vi "send&receive_multy_arrs.vi"() -> ()   [LabVIEW 2018, in "LV-Julia_ZMQ-Roundtrip_lib.lvlib"]
uses:
  LV-Julia_ZMQ-Roundtrip_lib.lvlib
  Server or client state.ctl
  detailed error info.ctl
  StackFrame.ctl
  Commands v2.ctl
  commands LV2Jl.ctl
  Julia functions enum.ctl
  0f3c6ff9-6efb-4048-9743-f0faf74ba571.vi
  1180a24e-9cfc-4814-956e-56f85e4fc15d.vi
  d2cb43a9-9305-42fb-ad58-bce983510195.vi
  4837e4b1-53a7-49b6-9aef-263877b89a45.vi
  5398bb44-7854-4704-a5a4-70900ab1788b.vi
  0f3c6ff9-6efb-4048-9743-f0faf74ba571.vi/a8133a9d-5cb4-4f45-826d-93f84bf6eb0d.vi
  0f3c6ff9-6efb-4048-9743-f0faf74ba571.vi/13f44d60-32a4-4ee7-b81c-21f7a391c3aa.vi
  0f3c6ff9-6efb-4048-9743-f0faf74ba571.vi/9f4fcee5-9fb3-4ec4-aeb1-d194e55cfefe.vi
  0f3c6ff9-6efb-4048-9743-f0faf74ba571.vi/1d479851-527b-4588-bf0b-60628e8bf317.vi
  0f3c6ff9-6efb-4048-9743-f0faf74ba571.vi/26ca6034-af2a-482b-8391-d55ce4957874.vi
  1180a24e-9cfc-4814-956e-56f85e4fc15d.vi/745acb1a-d655-4255-af81-9cf684133840.vi
  1180a24e-9cfc-4814-956e-56f85e4fc15d.vi/00973f5a-5f23-4306-b9aa-355ac52cfc45.vi
  1180a24e-9cfc-4814-956e-56f85e4fc15d.vi/c6eed95d-99c6-43df-958f-043b05f188e9.vi
  1180a24e-9cfc-4814-956e-56f85e4fc15d.vi/2e50c6a9-e645-434a-9e40-f73025a6ffce.vi
  1180a24e-9cfc-4814-956e-56f85e4fc15d.vi/339e4087-309e-456a-ab9d-330082cc7581.vi
  d2cb43a9-9305-42fb-ad58-bce983510195.vi/19be6d5a-1807-40f3-bdbe-1f3f52c696f0.vi
  d2cb43a9-9305-42fb-ad58-bce983510195.vi/aa24d0ac-04a8-4d7b-8f99-439a812d7bff.vi
  d2cb43a9-9305-42fb-ad58-bce983510195.vi/183daee5-84c7-4d39-a056-e1aa05b2b19e.vi
  4837e4b1-53a7-49b6-9aef-263877b89a45.vi/b7e14757-1b30-45b6-9c9e-f3055ae305b8.vi
  4837e4b1-53a7-49b6-9aef-263877b89a45.vi/187a7c1e-07ba-4c8d-9bdb-654d6cd0a580.vi
  5398bb44-7854-4704-a5a4-70900ab1788b.vi/24b2726a-72e9-4d38-b333-142c4ad70cae.vi
  5398bb44-7854-4704-a5a4-70900ab1788b.vi/ae670f7e-6490-4d67-937f-e0119a307e5a.vi
  0f3c6ff9-6efb-4048-9743-f0faf74ba571.vi/13f44d60-32a4-4ee7-b81c-21f7a391c3aa.vi/4fd0da60-a885-4f86-950c-51bd87ce8b7e.vi
  0f3c6ff9-6efb-4048-9743-f0faf74ba571.vi/9f4fcee5-9fb3-4ec4-aeb1-d194e55cfefe.vi/0c7f0749-4fca-4eec-9bb8-54480ed85867.vi
  0f3c6ff9-6efb-4048-9743-f0faf74ba571.vi/1d479851-527b-4588-bf0b-60628e8bf317.vi/c34eabd0-0321-4a17-ad95-65fcb7b0333a.vi
  1180a24e-9cfc-4814-956e-56f85e4fc15d.vi/00973f5a-5f23-4306-b9aa-355ac52cfc45.vi/cb92420a-3b20-40fb-957b-d1dd647802a0.vi
  1180a24e-9cfc-4814-956e-56f85e4fc15d.vi/c6eed95d-99c6-43df-958f-043b05f188e9.vi/f2a235e6-0b9e-43b4-b57c-a299a1c981e2.vi
  1180a24e-9cfc-4814-956e-56f85e4fc15d.vi/2e50c6a9-e645-434a-9e40-f73025a6ffce.vi/335e82b0-2764-49f6-958b-454fe2620a9a.vi
  4837e4b1-53a7-49b6-9aef-263877b89a45.vi/b7e14757-1b30-45b6-9c9e-f3055ae305b8.vi/13c95251-aaf3-4968-a2b1-71e97477a335.vi
  4837e4b1-53a7-49b6-9aef-263877b89a45.vi/b7e14757-1b30-45b6-9c9e-f3055ae305b8.vi/ab4a86bb-797d-4947-b82b-ab2adb434181.vi
  5398bb44-7854-4704-a5a4-70900ab1788b.vi/24b2726a-72e9-4d38-b333-142c4ad70cae.vi/167f8237-5b23-4042-87d7-597a2036b2c1.vi
  5398bb44-7854-4704-a5a4-70900ab1788b.vi/24b2726a-72e9-4d38-b333-142c4ad70cae.vi/addd60ed-eb33-4fa9-8646-f27a66fb9797.vi
  0f3c6ff9-6efb-4048-9743-f0faf74ba571.vi/13f44d60-32a4-4ee7-b81c-21f7a391c3aa.vi/4fd0da60-a885-4f86-950c-51bd87ce8b7e.vi/d91722bc-760f-488b-93ae-5bc6f1881f78.vi
  0f3c6ff9-6efb-4048-9743-f0faf74ba571.vi/9f4fcee5-9fb3-4ec4-aeb1-d194e55cfefe.vi/0c7f0749-4fca-4eec-9bb8-54480ed85867.vi/2bfc81f1-cfb7-4819-b1bc-540959743fb2.vi
  0f3c6ff9-6efb-4048-9743-f0faf74ba571.vi/1d479851-527b-4588-bf0b-60628e8bf317.vi/c34eabd0-0321-4a17-ad95-65fcb7b0333a.vi/b4dec757-f14e-4c32-8f18-a6a53eb12cfa.vi
  1180a24e-9cfc-4814-956e-56f85e4fc15d.vi/00973f5a-5f23-4306-b9aa-355ac52cfc45.vi/cb92420a-3b20-40fb-957b-d1dd647802a0.vi/e8ebe7f7-f03d-49ec-9fb8-d4a1a45a4ade.vi
  1180a24e-9cfc-4814-956e-56f85e4fc15d.vi/c6eed95d-99c6-43df-958f-043b05f188e9.vi/f2a235e6-0b9e-43b4-b57c-a299a1c981e2.vi/36ca0de6-0589-4a03-972d-fca6fdad2387.vi
  1180a24e-9cfc-4814-956e-56f85e4fc15d.vi/2e50c6a9-e645-434a-9e40-f73025a6ffce.vi/335e82b0-2764-49f6-958b-454fe2620a9a.vi/0d9d3acc-8ad3-4eff-83fb-bef53c6a881b.vi
  4837e4b1-53a7-49b6-9aef-263877b89a45.vi/b7e14757-1b30-45b6-9c9e-f3055ae305b8.vi/13c95251-aaf3-4968-a2b1-71e97477a335.vi/50b08b95-f687-4883-9b5c-2995c4691fc2.vi
  5398bb44-7854-4704-a5a4-70900ab1788b.vi/24b2726a-72e9-4d38-b333-142c4ad70cae.vi/167f8237-5b23-4042-87d7-597a2036b2c1.vi/0c43e3ab-dc7e-44be-9e5a-46602dd1e47d.vi
  0f3c6ff9-6efb-4048-9743-f0faf74ba571.vi/13f44d60-32a4-4ee7-b81c-21f7a391c3aa.vi/4fd0da60-a885-4f86-950c-51bd87ce8b7e.vi/d91722bc-760f-488b-93ae-5bc6f1881f78.vi/81bb06db-bbc8-4c4f-bf8c-0a9139f35f47.vi
  0f3c6ff9-6efb-4048-9743-f0faf74ba571.vi/9f4fcee5-9fb3-4ec4-aeb1-d194e55cfefe.vi/0c7f0749-4fca-4eec-9bb8-54480ed85867.vi/2bfc81f1-cfb7-4819-b1bc-540959743fb2.vi/ceb014c5-17c5-4aee-87b4-bdb5202f11bf.vi
  0f3c6ff9-6efb-4048-9743-f0faf74ba571.vi/1d479851-527b-4588-bf0b-60628e8bf317.vi/c34eabd0-0321-4a17-ad95-65fcb7b0333a.vi/b4dec757-f14e-4c32-8f18-a6a53eb12cfa.vi/3b214c27-556c-42a7-8fef-6ab7ffc3abfe.vi
  1180a24e-9cfc-4814-956e-56f85e4fc15d.vi/00973f5a-5f23-4306-b9aa-355ac52cfc45.vi/cb92420a-3b20-40fb-957b-d1dd647802a0.vi/e8ebe7f7-f03d-49ec-9fb8-d4a1a45a4ade.vi/a50604c4-b02c-41aa-8651-ec1557e36820.vi
  1180a24e-9cfc-4814-956e-56f85e4fc15d.vi/c6eed95d-99c6-43df-958f-043b05f188e9.vi/f2a235e6-0b9e-43b4-b57c-a299a1c981e2.vi/36ca0de6-0589-4a03-972d-fca6fdad2387.vi/17266f24-6c92-4fe0-b395-2dcbb4c32836.vi
  1180a24e-9cfc-4814-956e-56f85e4fc15d.vi/2e50c6a9-e645-434a-9e40-f73025a6ffce.vi/335e82b0-2764-49f6-958b-454fe2620a9a.vi/0d9d3acc-8ad3-4eff-83fb-bef53c6a881b.vi/8f1dd33f-3a61-4420-ad07-afe7428103ca.vi
  check ID validity.vi
  bindata_descr to JSON.vi
  convert Jl functions enum to string.vi
  check cluster field names.vi
  concat JSON.vi
  <vilib>/Utility/error.llb/Error Cluster From Error Code.vi
panel:
  out "U64arr":u64[](array[numeric])
  out "arrays equal":bool
  out "elems equal":bool
  in  "next":bool
  in  "stop LV only":bool
  in  "stop":bool
  out "detailed error info":T1
  out "elem sent":sgl
  out "elem received":dbl
  out "testarr":sgl[][](array[numeric])
  in  "index to return":cluster{"idx":u16[]}={"idx"=[3, 4, 1]} {"idx" min=1}
  out "Jl Server state out":T3
  out "short err code":u8
  out "final error":errorcluster
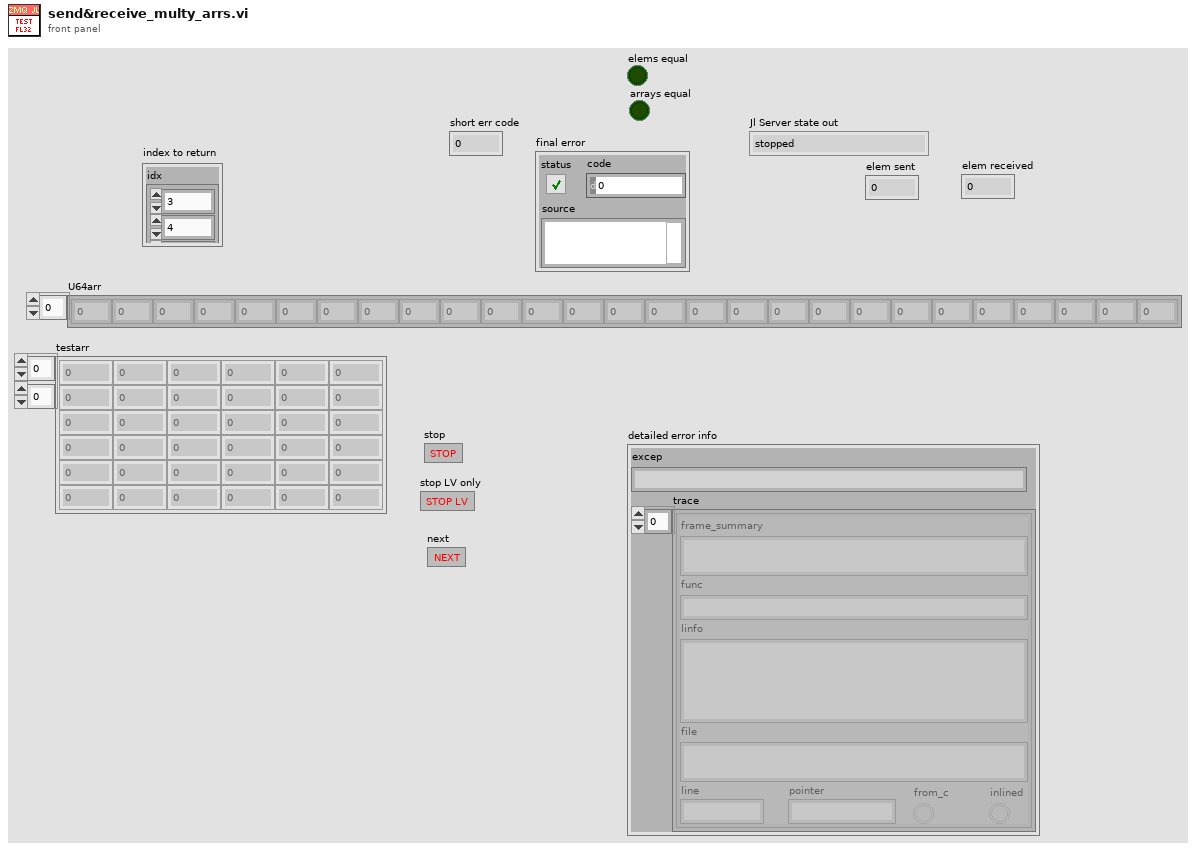
[diagram p1: front panel]
types:
  T1 = typedef "LV-Julia_ZMQ-Roundtrip_lib.lvlib/detailed error info.ctl" = cluster{"excep":string, "trace":T2[]}
  T2 = typedef "LV-Julia_ZMQ-Roundtrip_lib.lvlib/StackFrame.ctl" = cluster{"frame_summary":string, "func":string, "linfo":string, "file":string, "line":i32, "pointer":u64, "from_c":bool, "inlined":bool}
  T3 = typedef "LV-Julia_ZMQ-Roundtrip_lib.lvlib/Server or client state.ctl" = enum16{"stopped", "running", "unknown"}
  T4 = typedef "LV-Julia_ZMQ-Roundtrip_lib.lvlib/Commands v2.ctl" = enum16{"Start Jl-server & Init LV-client", "Send request & Get response ", "Stop Jl-server & Cleanup LV-client", "Cleanup LV-client", "Start Jl-server", "Stop Jl-server", "Init LV-Client", "Cleanup LV-Client", "(not allowed)", "Set LV Client state", "Set Jl Server state"}
  T5 = typedef "LV-Julia_ZMQ-Roundtrip_lib.lvlib/Julia functions enum.ctl" = enum16{"myf1", "myf2", "myf3", "test_bin2nums", "test_rgbimg", "numarr_loopback", "numarrs_lpbk", "Not_a_Fun"}
  T6 = typedef "commands LV2Jl.ctl" = u8
  T7 = typedef "Bindata&description.ctl" = cluster{"bindata_descr":T8[], "bindata":u8[]}
  T8 = typedef "LV-Julia_ZMQ-Roundtrip_lib.lvlib/Bindata description.ctl" = cluster{"nofbytes":i32, "numtype":string, "start":i32, "arrdims":i32[], "kwarg_name":string, "category":string}
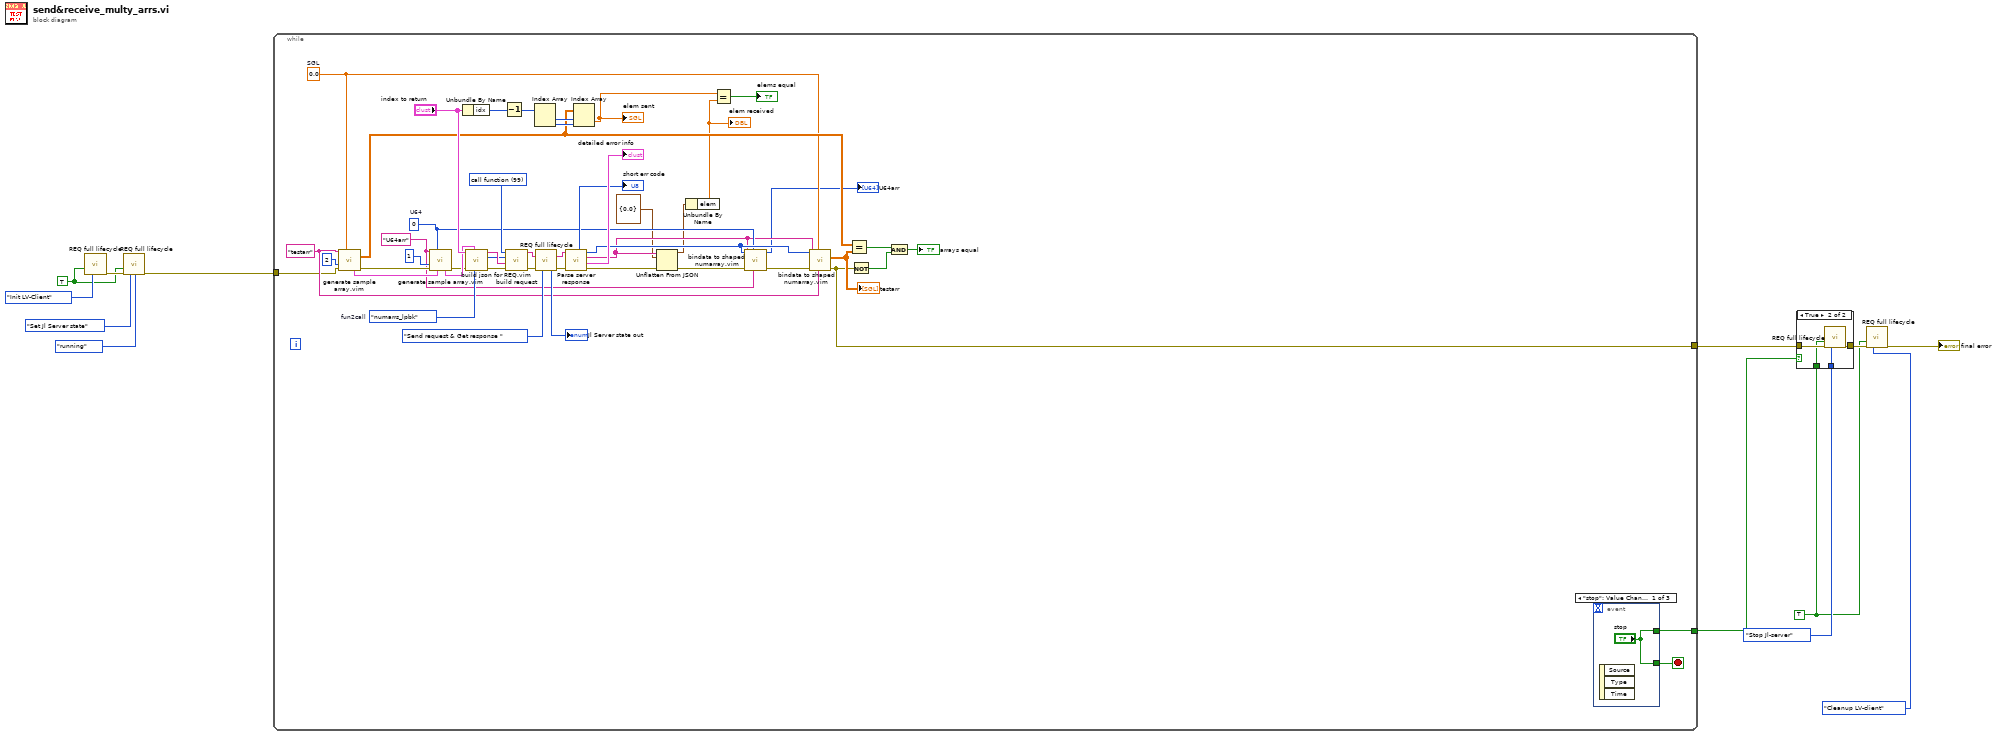
[diagram p0: block diagram]
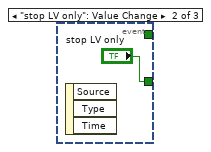
[diagram p2: hidden frame]
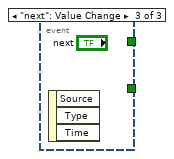
[diagram p3: hidden frame]
diagram:
  w4 = TRUE ("Force command")
  w8 = TRUE ("Force command")
  n1 = call "REQ full lifecycle.vi"("Force command"=w4, "command"=Commands_v2."Init LV-Client") -> ("error out"=w6:errorcluster)  [unwired: 10 in, 3 out]
  n2 = call "REQ full lifecycle.vi"("Force command"=w4, "error in"=w6, "command"=Commands_v2."Set Jl Server state", "Jl Server state in"=Server_or_client_state."running") -> ("error out"=w2:errorcluster)  [unwired: 8 in, 3 out]
  n3 = while {
    tunnel: w2 -> [w40]
    tunnel: [w32] -> w13
    tunnel: [w35] -> w1
    stop <- w36 stop-if-true
    w19 = "U64arr" ("kwarg_name")
    w21 = u64 0  # U64
    w29 = sgl 0.0  # SGL
    w54 = Julia_functions_enum."numarrs_lpbk"  # fun2call
    w47 = "testarr" ("Tag")
    w55 = T6 99 items=["call function"=99, "ping"=112, "stop"=115] ("Command")
    n4 = call "generate sample array.vim"("kwarg_name"=w47, "type"=w29, "dims"=2 ("arr1 dimension"), "error in (no error)"=w40) -> ("Array 2D"=w31:sgl[][], "Bindata & descr out"=w28:T7, "error out"=w26:errorcluster)  [unwired: 5 in, 4 out]
    n5 = call "generate sample array.vim"("kwarg_name"=w19, "type"=w21, "dims"=u8 1, "error in (no error)"=w26, "Bindata & descr in"=w28) -> ("Bindata & descr out"=w27:T7, "error out"=w25:errorcluster)  [unwired: 4 in, 5 out]
    n6 = Unbundle By Name("index to return") -> ("idx"=w44:u16[])
    n7 = call "build json for REQ.vim"("fun2call"=w54, "Bindata & descr in"=w27, "error in (no error)"=w25, "Arguments 1"="index to return") -> ("error out"=w60:errorcluster, "bindata out"=w49:u8[], "JSON string out"=w50:string)  [unwired: 5 in]
    n8 = Decrement(x=w44) -> (x-1=w43:u16[])
    n9 = call "build request.vi"("error in (no error)"=w60, "JSON data"=w50, "binary data"=w49, "Command"=w55) -> ("error out"=w58:errorcluster, "REQ string"=w59:string)  [unwired: 6 in]
    n10 = Index Array(array=w43) -> (element #1=w38:u16, element #2=w37:u16)  [unwired: 2 in]
    n11 = call "REQ full lifecycle.vi"("data to send"=w59, "error in"=w58, "command"=Commands_v2."Send request & Get response ") -> ("server response"=w52:string, "Jl Server state out"=→"Jl Server state out":T3, "error out"=w57:errorcluster)  [unwired: 9 in, 1 out]
    n12 = call "Parse server response.vi"("error in (no error)"=w57, "server response in"=w52) -> ("error out"=w45:errorcluster, "detailed error info"=→"detailed error info":T1, "JSON out"=w20:string, "binary data"=w24:u8[], "return code"=→"short err code":u8)  [unwired: 3 in, 2 out]
    n13 = Index Array(array=w31, index (row)=w38, index (col)=w37) -> (element=w42:sgl)
    "elem sent" <- w42
    n14 = Unflatten From JSON(JSON string=w20, type and defaults=cluster{"elem":dbl} {"elem"=0.0} ("parsed response"), error in (no error)=w45) -> (value=w15:cluster{"elem":dbl}, error out=w17:errorcluster)  [unwired: 4 in]
    n15 = Unbundle By Name(w15) -> ("elem"=w14:dbl)
    "elem received" <- w14
    n16 = Equal?(x=w42, y=w14) -> (x = y?=→"elems equal":bool)
    n17 = call "bindata to shaped numarray.vim"("kwarg_name"=w19, "data type"=w21, "error in (no error)"=w17, "bindata_descr"=w20, "binary data"=w24) -> ("error out"=w23:errorcluster, "numarray 1D"=→"U64arr":u64[])  [unwired: 3 in, 2 out]
    n18 = call "bindata to shaped numarray.vim"("kwarg_name"=w47, "data type"=w29, "error in (no error)"=w23, "bindata_descr"=w20, "binary data"=w24) -> ("error out"=w32:errorcluster, "numarray 2D"=w46:sgl[][])  [unwired: 3 in, 2 out]
    "testarr" <- w46
    n19 = Equal?(x=w31, y=w46) -> (x = y?=w33:bool)
    n20 = Not(x=w32) -> (.not. x?=w34:bool)
    n21 = And(x=w33, y=w34) -> (x .and. y?=→"arrays equal":bool)
    n22 = event shown="[0] \"stop\": Value Change" {
      selector: _ -> [_ _ _]
      dyn-events: _ -> [_ _ _]
      timeout: _ -> [_ _ _]
      tunnel: ["stop" "stop LV only" _] -> w36
      tunnel: ["stop" _ _] -> w35
      event "stop": Value Change {
        n23 = event-data() -> ()  [unwired: 1 in, 3 out]
      }
      event "stop LV only": Value Change {
        n24 = event-data() -> ()  [unwired: 1 in, 3 out]
      }
      event "next": Value Change {
        n25 = event-data() -> ()  [unwired: 1 in, 3 out]
      }
    }
  }
  n26 = case shown="True" w1 {
    tunnel: w13 -> [w64 w68]
    tunnel: Commands_v2."Stop Jl-server" ("command") -> [_ w67]
    tunnel: [w64 w66] -> w11
    tunnel: w8 -> [_ w65]
    frame False {
    }
    frame True {
      n27 = call "REQ full lifecycle.vi"("Force command"=w65, "error in"=w68, "command"=w67) -> ("error out"=w66:errorcluster)  [unwired: 9 in, 3 out]
    }
  }
  n28 = call "REQ full lifecycle.vi"("Force command"=w8, "error in"=w11, "command"=Commands_v2."Cleanup LV-client") -> ("error out"=→"final error":errorcluster)  [unwired: 9 in, 3 out]
